vi "Get LogEngine RawDataQs.vi"(8 "error in (no error)":errorcluster, 11 "LogEngine":refnum<class "LogEngine.lvclass">) -> (0 "error out":errorcluster, 2 "LogEngine DataQs":T1, 3 "LogEngine out":refnum<class "LogEngine.lvclass">)   [LabVIEW 2017]
uses:
  LogEngine.lvclass
  DAQ/Process/ProcessSupport/TD local raw AI Data--cluster.ctl
  DAQ/DAQ.lvclass
  Data Types/TD Queues_LogEngine.ctl
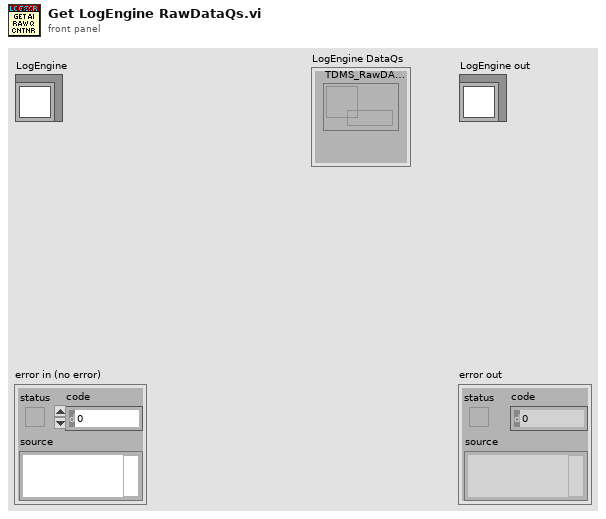
[diagram p1: front panel]
types:
  T1 = typedef "TD Queues_LogEngine.ctl" = cluster{"TDMS_RawDAQDataQ":refnum<queue>}
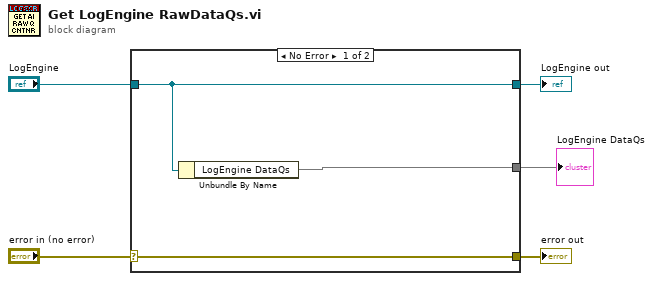
[diagram p0: block diagram]
diagram:
  n1 = case shown="No Error" "error in (no error)" {
    selector: "error in (no error)" -> [w8 w9]
    tunnel: [w8 w9] -> w4
    tunnel: [w7 w10] -> w2
    tunnel: "LogEngine" -> [w7 w10]
    tunnel: [w6 _] -> w1
    frame No Error {
      n2 = Unbundle By Name(w7) -> ("LogEngine DataQs"=w6)
    }
    frame Error {
    }
  }
  "error out" <- w4
  "LogEngine out" <- w2
  "LogEngine DataQs" <- w1
